vi "SubPanel_Size and Insert.vi"(6 "Border Spacing":i32=-2, 7 "VI":refnum<vi>, 8 "Error":errorcluster, 9 "Frame Ref":refnum<vi>, 11 "Sub Panel":refnum<vi>) -> (0 "Error Out":errorcluster, 1 "Vi Inserted Out":bool, 2 "Success Out":bool, 3 "Sub Panel 2":refnum<vi>)   [LabVIEW 2015]
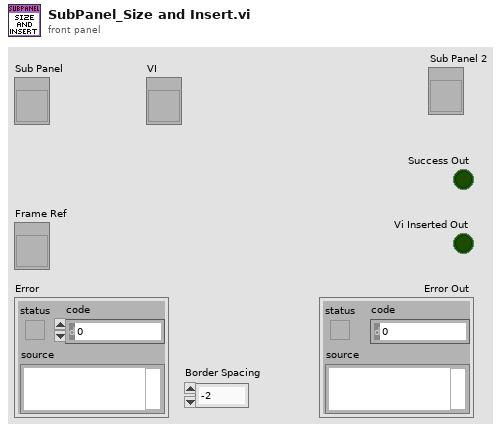
[diagram p1: front panel]
types:
  T1 = typedef "LVRectTypeDef.ctl" = cluster{"Left":i16, "Top":i16, "Right":i16, "Bottom":i16}
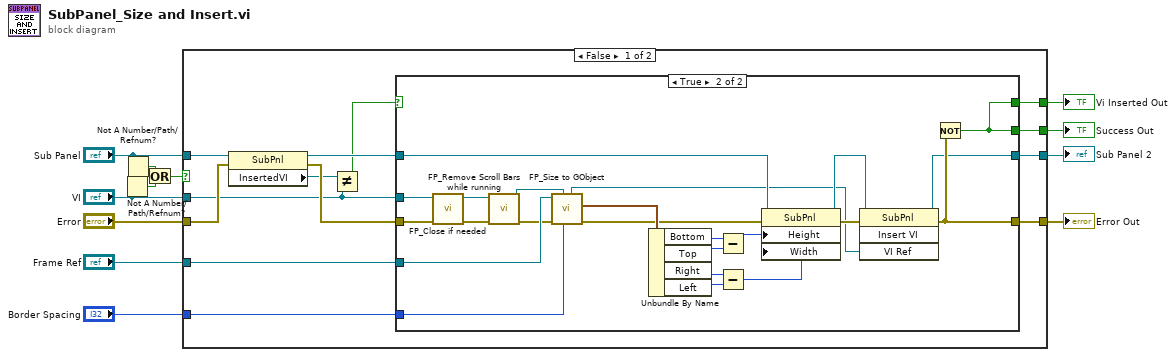
[diagram p0: block diagram]
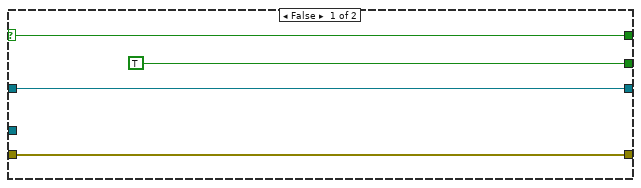
[diagram p2: hidden frame]
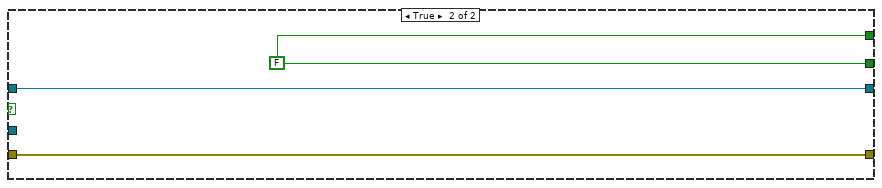
[diagram p3: hidden frame]
diagram:
  n1 = Not A Number/Path/Refnum?(number/path/refnum="VI") -> (NaN/Path/Refnum?=w9:bool)
  n2 = Not A Number/Path/Refnum?(number/path/refnum="Sub Panel") -> (NaN/Path/Refnum?=w10:bool)
  n3 = Or(x=w10, y=w9) -> (x .or. y?=w7:bool)
  n4 = case shown="False" w7 {
    tunnel: [w25 w54] -> w12
    tunnel: "Error" -> [w23 w55]
    tunnel: "Sub Panel" -> [w19 w53]
    tunnel: "VI" -> [w18 _]
    tunnel: [w17 w55] -> w8
    tunnel: [w16 w54] -> w6
    tunnel: "Frame Ref" -> [w15 _]
    tunnel: [w14 w53] -> w4
    tunnel: "Border Spacing" -> [w13 _]
    frame False {
      n5 = property class="SubPnl"(reference=w19, error in=w23) -> (reference out=w24:refnum<vi>, error out=w22:errorcluster, "InsertedVI"=w21:refnum<vi>)
      n6 = Not Equal?(x=w21, y=w18) -> (x != y?=w20:bool)
      n7 = case shown="True" w20 {
        selector: w20 -> [w27 _]
        tunnel: [w28 w44] -> w17
        tunnel: [TRUE w42] -> w25
        tunnel: w24 -> [w26 w43]
        tunnel: w22 -> [w28 w39]
        tunnel: w18 -> [_ w40]
        tunnel: [w27 w42] -> w16
        tunnel: w15 -> [_ w33]
        tunnel: [w26 w41] -> w14
        tunnel: w13 -> [_ w30]
        frame False {
        }
        frame True {
          n8 = call "FP_Close if needed.vi"("Error"=w39, "VI"=w40) -> ("Error Out"=w37:errorcluster, "VI Out"=w38:refnum<vi>)  [unwired: 8 in]
          n9 = call "FP_Remove Scroll Bars while running.vi"("Error"=w37, "VI"=w38) -> ("Error Out"=w32:errorcluster, "VI Out"=w34:refnum<vi>)  [unwired: 8 in]
          n10 = call "FP_Size to GObject.vi"("Border Spacing (2 Px)"=w30, "Calling VI's Ref"=w34, "Error"=w32, "GObj Refnum"=w33) -> ("Error Out"=w31:errorcluster, "Front Panel.PanelBounds Out"=w36:T1, "Calling VI's Ref Out"=w35:refnum<vi>)  [unwired: 2 in, 3 out]
          n11 = Unbundle By Name(w36) -> ("Bottom"=w46:i16, "Top"=w47:i16, "Right"=w48:i16, "Left"=w49:i16)
          n12 = Subtract(x=w46, y=w47) -> (x-y=w50:i16)
          n13 = Subtract(x=w48, y=w49) -> (x-y=w51:i16)
          n14 = property class="SubPnl"(reference=w43, error in=w31, "Height"=w50, "Width"=w51) -> (reference out=w45:refnum<vi>, error out=w52:errorcluster)
          n15 = invoke class="SubPnl" method="Insert VI"(reference=w45, error in=w52, "VI Ref"=w35) -> (reference out=w41:refnum<vi>, error out=w44:errorcluster)  [unwired: 1 in, 2 out]
          n16 = Not(x=w44) -> (.not. x?=w42:bool)
        }
      }
    }
    frame True {
      w54 = FALSE
    }
  }
  "Success Out" <- w12
  "Error Out" <- w8
  "Vi Inserted Out" <- w6
  "Sub Panel 2" <- w4
